vi "Close.vi"(8 "error in (no error)":errorcluster, 11 "Comm Protocol in":refnum<class "Comm Protocol.lvclass">) -> (0 "error out":errorcluster, 3 "Comm Protocol out":refnum<class "Comm Protocol.lvclass">)   [LabVIEW 2021, in "Comm Protocol.lvclass"]
uses:
  Comm Protocol.lvclass
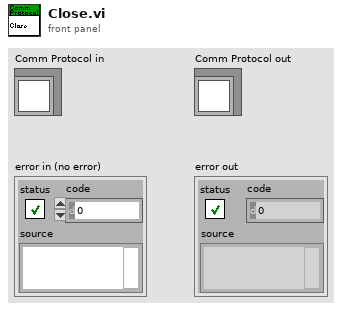
[diagram p1: front panel]
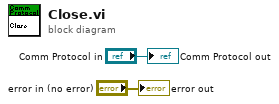
[diagram p0: block diagram]
diagram:
  "error out" <- "error in (no error)"
  "Comm Protocol out" <- "Comm Protocol in"
